vi "Make Time Stamp File Path.vi"(8 "t0":timestamp, 11 "base path":path) -> (3 "file path":path)   [LabVIEW 2023]
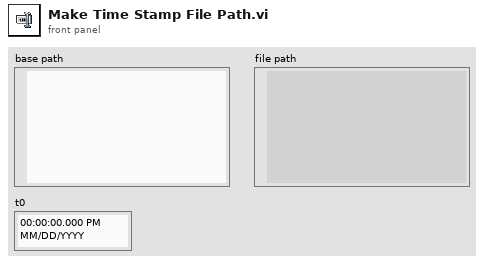
[diagram p1: front panel]
types:
  T1 = typedef "LVDateTimeRec.ctl" = cluster{"fractional second":dbl, "second":i32, "minute":i32, "hour":i32, "day of month":i32, "month":i32, "year":i32, "day of week":i32, "day of year":i32, "DST":i32}
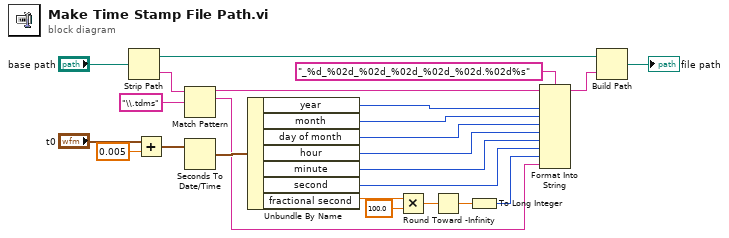
[diagram p0: block diagram]
diagram:
  n1 = Strip Path(path="base path") -> (stripped path=w22:path, name=w21:string)
  n2 = Add(x="t0", y=0.005) -> (x+y=w2:timestamp)
  n3 = Match Pattern(string=w21, regular expression="\\.tdms") -> (before substring=w17:string, match substring=w15:string)  [unwired: 1 in, 2 out]
  n4 = Seconds To Date/Time(time stamp (now)=w2) -> (date time rec=w18:T1)  [unwired: 1 in]
  n5 = Unbundle By Name(w18) -> ("year"=w13:i32, "month"=w12:i32, "day of month"=w11:i32, "hour"=w10:i32, "minute"=w9:i32, "second"=w8:i32, "fractional second"=w7:dbl)
  n6 = Multiply(x=w7, y=100.0) -> (x*y=w5:dbl)
  n7 = Round Toward -Infinity(1:w5) -> (0:w4:dbl)
  n8 = To Long Integer(number=w4) -> (32bit integer=w3:i32)
  n9 = Format Into String(format string="_%d_%02d_%02d_%02d_%02d_%02d.%02d%s", initial string=w17, w13, w12, w11, w10, w9, w8, w3, w15) -> (resulting string=w14:string)  [unwired: 1 in, 1 out]
  n10 = Build Path(base path=w22, name or relative path=w14) -> (appended path=→"file path":path)
